vi "PCert-Container-AskActor.vi"(8 "error in (no error)":errorcluster, 9 "Ask Payload":string, 10 "Ask Command":string="Shut Up!", 11 "ERP-Container-UI in":refnum<class "PCert-Container-UI.lvclass">) -> (0 "error out":errorcluster, 2 "Response Header":string, 3 "ERP-Container-UI out":refnum<class "PCert-Container-UI.lvclass">)   [LabVIEW 2013, in "PCert-Container-UI.lvclass"]
uses:
  PCert-Container-UI.lvclass
  PCert-Container-UI.lvclass/PCert-Container-UI.ctl
  ftw-dataflow/Actor/src/Connector/FTW-ActorConnector.lvclass
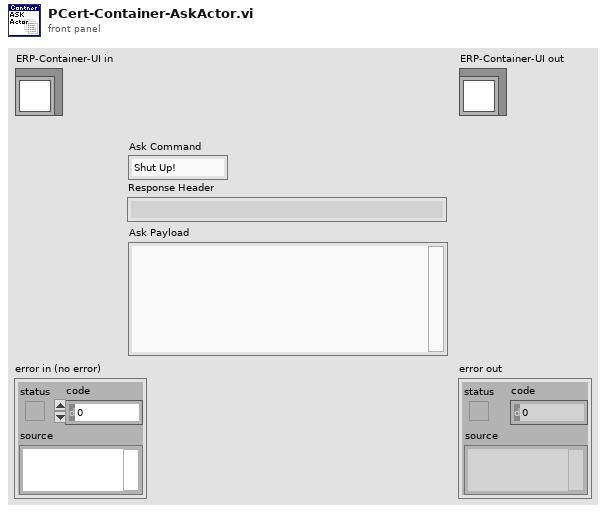
[diagram p1: front panel]
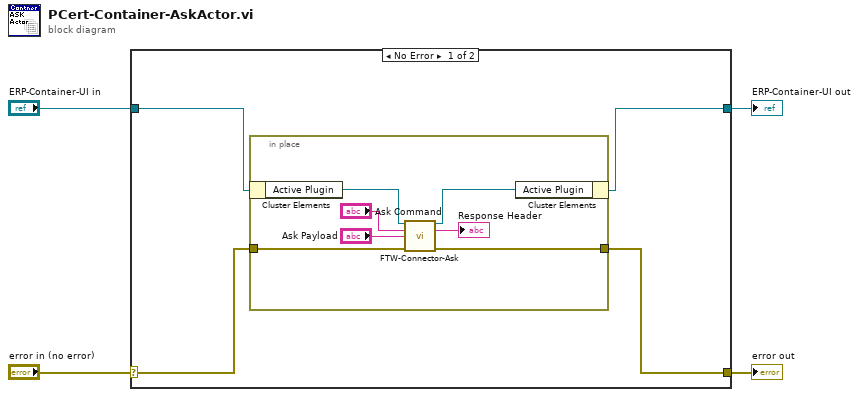
[diagram p0: block diagram]
diagram:
  n1 = case shown="No Error" "error in (no error)" {
    selector: "error in (no error)" -> [w8 w17]
    tunnel: [w7 w17] -> w3
    tunnel: [w5 w16] -> w1
    tunnel: "ERP-Container-UI in" -> [w6 w16]
    frame No Error {
      n2 = in-place {
        in-place-border: w8 -> [w11]
        in-place-border: [w10] -> w7
        n3 = in-place-cluster #1(w6) -> ("Active Plugin"=w15:refnum<class "FTW-ActorConnector.lvclass">)
        n4 = call "FTW-Connector-Ask.vi"("FTW Actor Connector"=w15, "Request Header"="Ask Command", "Request Body"="Ask Payload", "error in"=w11) -> ("FTW Actor Connector out"=w14:refnum<class "FTW-ActorConnector.lvclass">, "Response Header"=→"Response Header":string, "error out"=w10:errorcluster)  [unwired: 7 in, 2 out]
        n5 = in-place-cluster #1("Active Plugin"=w14) -> (w5:refnum<class "PCert-Container-UI.lvclass">)
      }
    }
    frame Error {
    }
  }
  "error out" <- w3
  "ERP-Container-UI out" <- w1
